vi "MapLineareinheit.vi"(0 "InputArray":dbl[][](array[numeric])=array200x300[60000 elements], 5 "aktuelle z(cm)":dbl=100.0, 7 "aktuelle x(c m)":dbl=117.29768886687648, 9 "höhe":dbl=0.5) -> (8 "OutputArray":dbl[][](array[numeric]), 15 "Map_Lineareinheit":dbl[][](graph))   [LabVIEW 2014]
panel:
  out "Anzahl x  Elemente":i32=200
  out "Anzahl y Elemente":i32=300
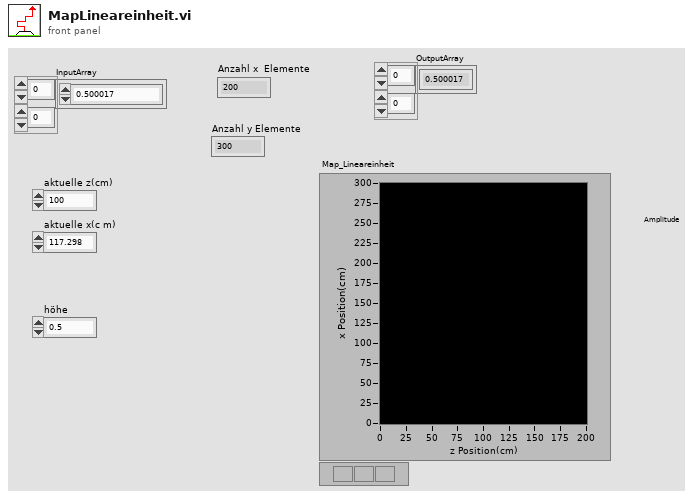
[diagram p1: front panel]
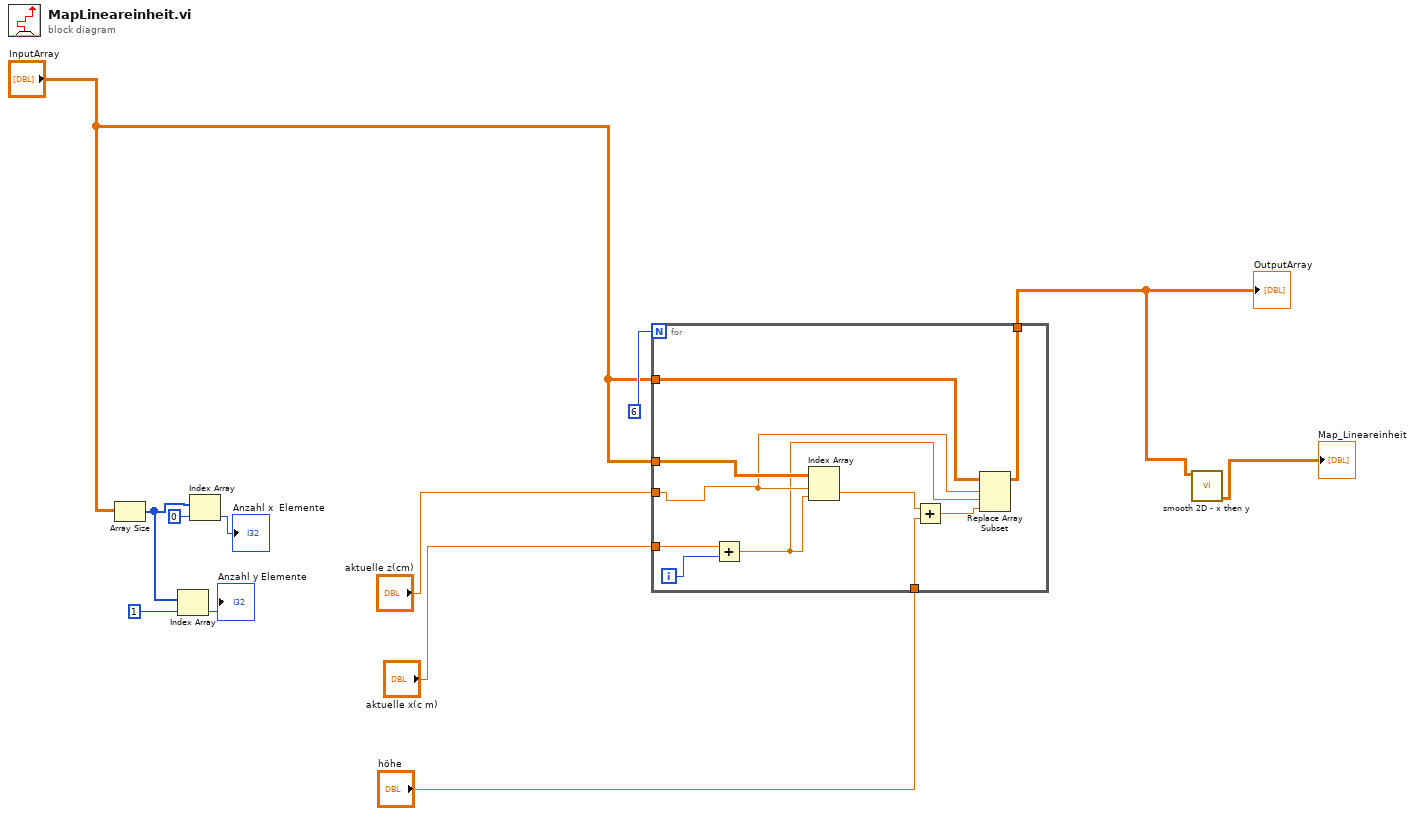
[diagram p0: block diagram]
diagram:
  n1 = Array Size(array="InputArray") -> (size(s)=w9:i32[])
  n2 = Index Array(array=w9, index=1 ("Index")) -> (element=→"Anzahl y Elemente":i32)
  n3 = Index Array(array=w9, index=0 ("Index")) -> (element=→"Anzahl x  Elemente":i32)
  n4 = for {
    N: 6 -> [_]
    tunnel: "InputArray" -> [w22]
    tunnel: "aktuelle z(cm)" -> [w16]
    tunnel: "aktuelle x(c m)" -> [w21]
    tunnel: "InputArray" -> [w17]
    tunnel: "höhe" -> [w18]
    tunnel: [w13] -> w2
    i -> [w20]
    n5 = Add(x=w21, y=w20) -> (x+y=w15:dbl)
    n6 = Index Array(array=w22, index (row)=w16, index (col)=w15) -> (element=w19:dbl)
    n7 = Add(x=w19, y=w18) -> (x+y=w14:dbl)
    n8 = Replace Array Subset(array=w17, new element=w14, index (row)=w16, index (col)=w15) -> (w13:dbl[][])
  }
  "OutputArray" <- w2
  n9 = call "smooth 2D - x then y.vi"("2D array"=w2) -> ("x+y"=→"Map_Lineareinheit":dbl[][])  [unwired: 10 in]
